vi "crio_FPGA_encoder.vi"() -> ()   [LabVIEW 2019]
uses:
  <vilib>/rvi/Emulation/niFpgaSctlEmulationGetInTimedLoop.vi
  <vilib>/rvi/Emulation/niFpgaProcessEmulError.vi
  <vilib>/rvi/eio/common/nirviEmuTemplateMethod_errors.vi
  <vilib>/rvi/Emulation/niFpgaGetClockAttributes.vi
  <vilib>/rvi/Emulation/niFpgaEmulationReportErrorSimple.vi
  <vilib>/rvi/Emulation/niFpgaCriticalErrorInLSC.vi
  <vilib>/eio/EIOMethodNode/EIOMethodNode.xnode
  <vilib>/eio/EIONode/EIONode.xnode
panel:
  in  "stop":bool
  in  "Encoder Debug":bool
  in  "Loop Timer DAQ":u32=1 caption="Loop Time(uSec)"
  in  "Position Reset":bool
  out "Position (Counts)":i64
  out "B":bool
  out "A":bool
  out "B'":bool
  out "A'":bool
  in  "Velocity Interval (uSec)":u32=1000
  out "Acceleration (Counts/Interval)":i32
  out "Velocity (Counts/Interval)":i32
  out "ConnectorA/DIO13":bool
  out "ConnectorA/DIO12":bool
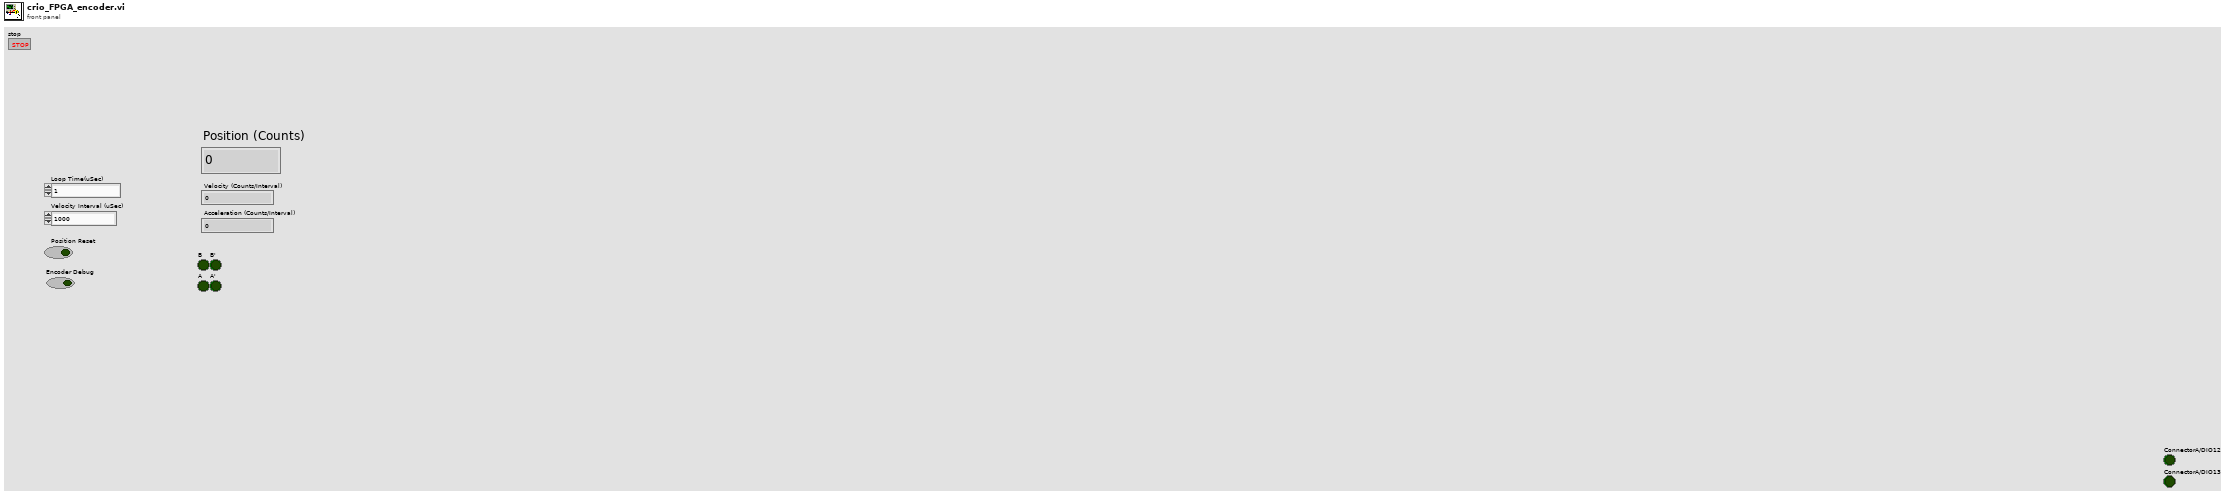
[diagram p1: front panel]
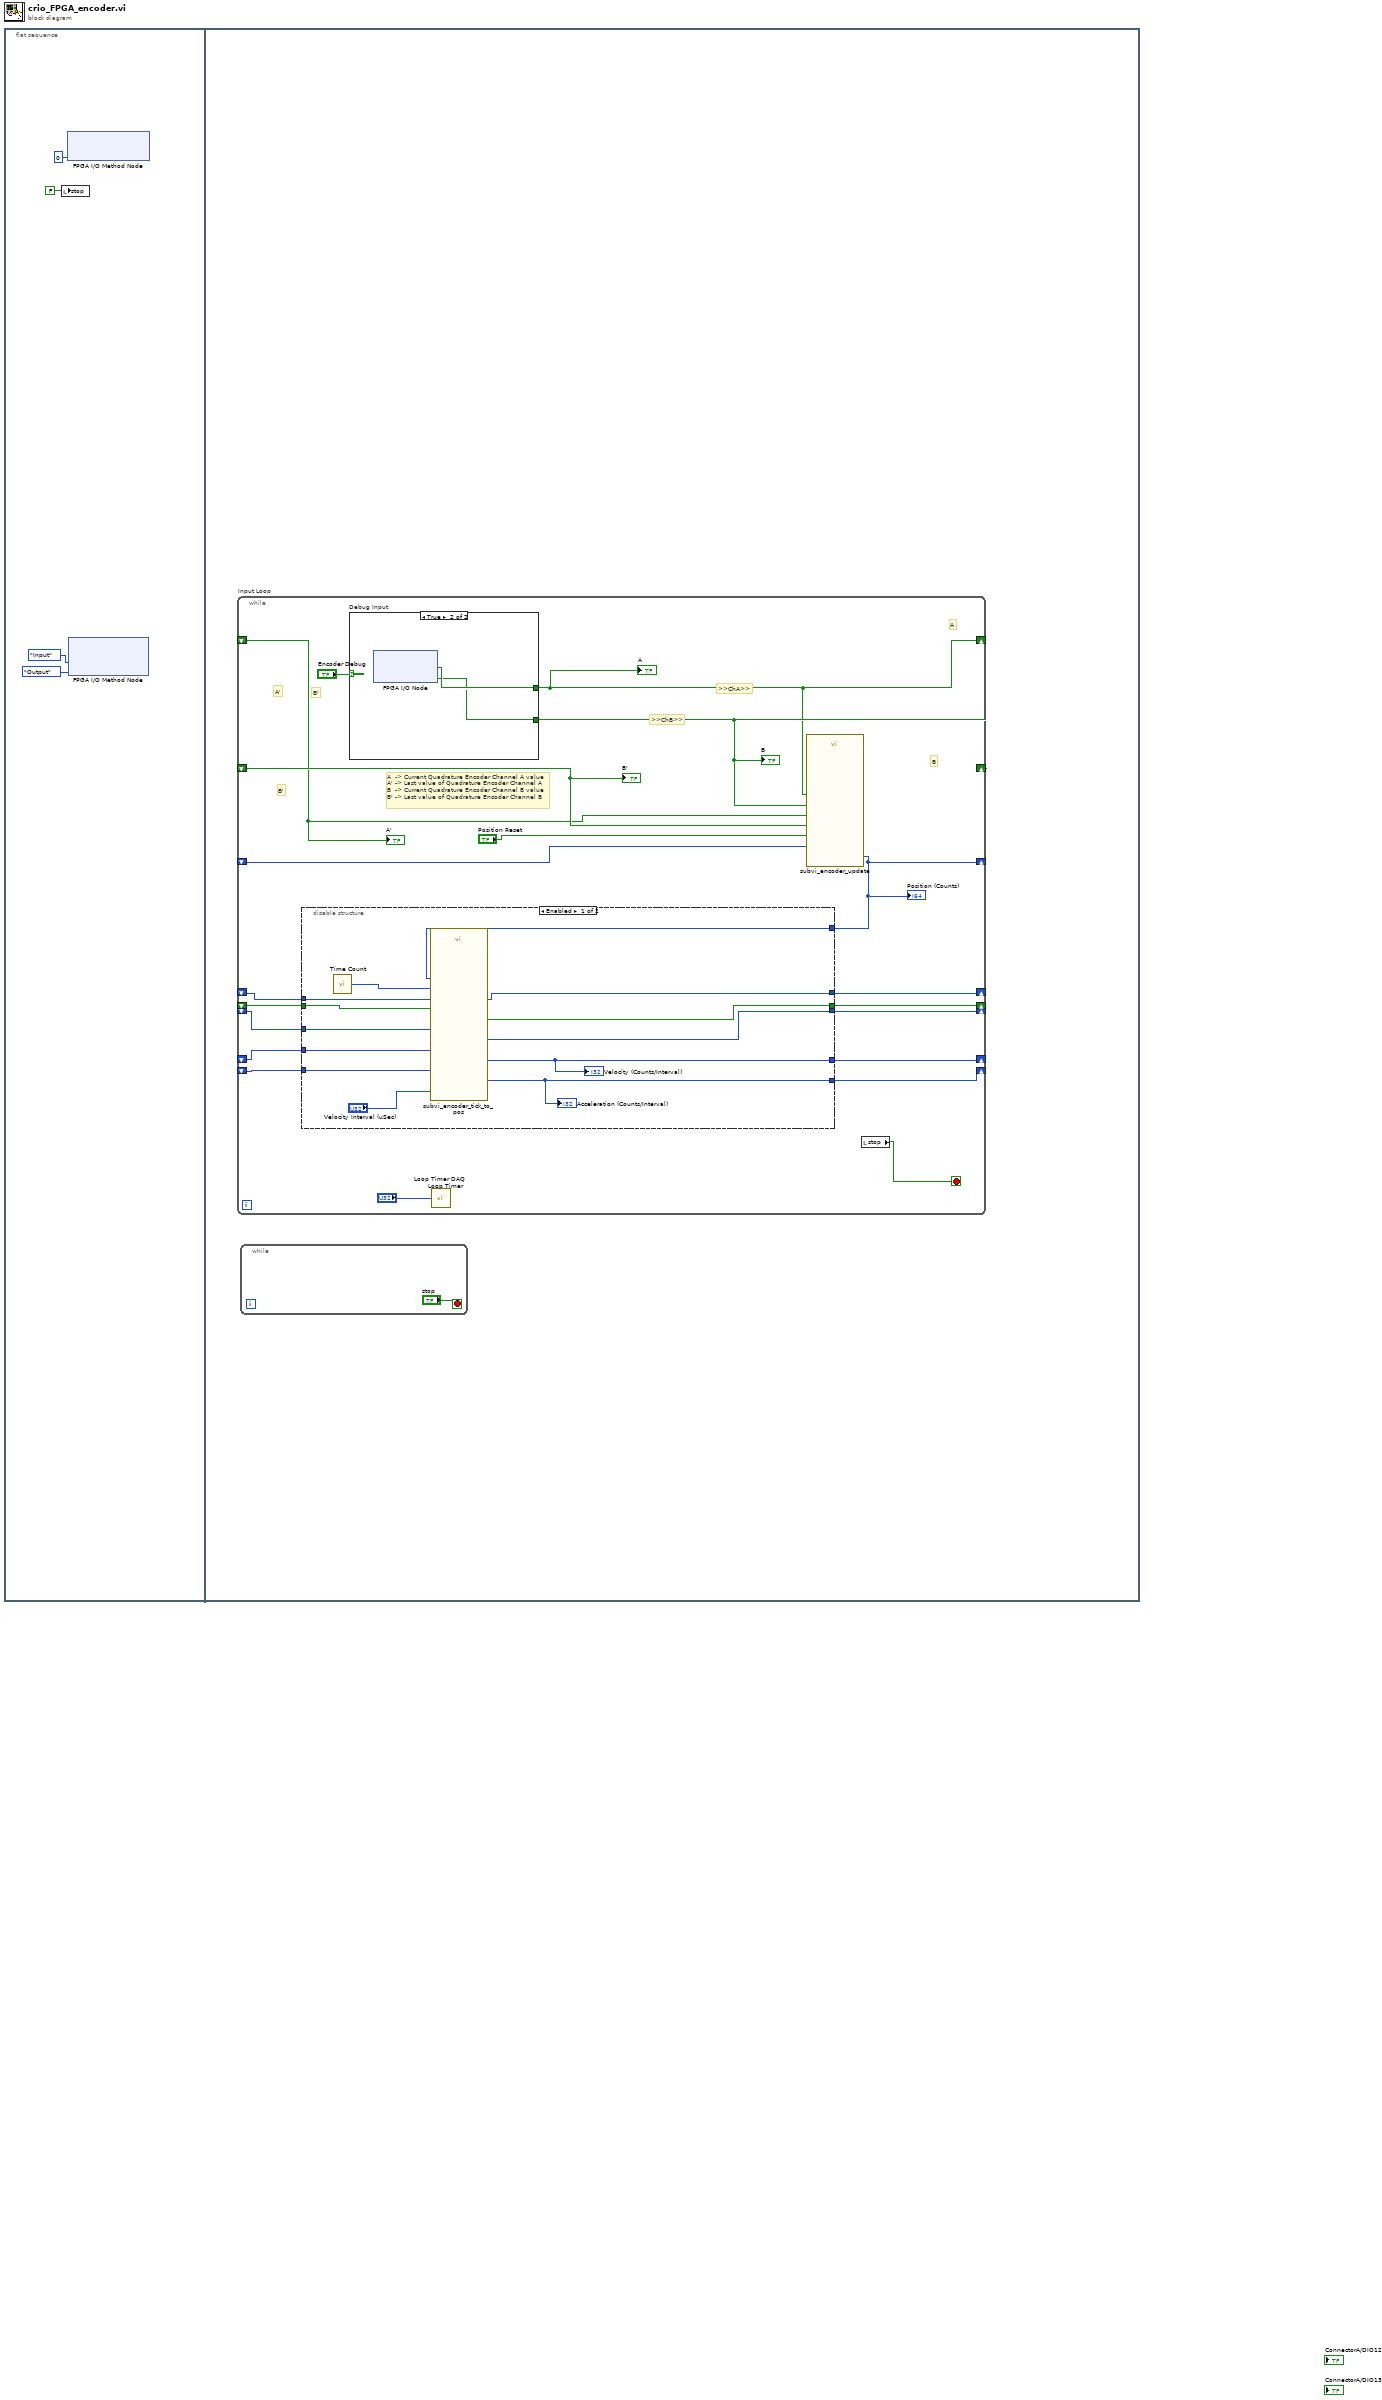
[diagram p0: block diagram]
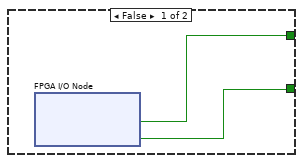
[diagram p3: hidden frame]
diagram:
  n1 = flat-sequence {
    frame #0 {
      n2 = local write "stop"(FALSE ("stop")) -> ()
      n3 = xnode "FPGA I/O Method Node"("Enable"=u8 0) -> ()  [unwired: 1 in, 1 out]
      n4 = xnode "FPGA I/O Method Node"("DIO 7:4"=enum8{"No Change", "Input", "Output"}."Input", "DIO 3:0"=enum8{"No Change", "Input", "Output"}."Output") -> ()  [unwired: 1 in, 1 out]
    }
    frame #1 {
      n5 = while "Input Loop" {
        shift-right: [w19] -> _
        shift-left: _ -> [w22]
        shift-right: [w18] -> _
        shift-left: _ -> [w21]
        shift-right: [w14] -> _
        shift-left: _ -> [w20]
        shift-right: [w7] -> _
        shift-left: _ -> [w17]
        shift-right: [w8] -> _
        shift-left: _ -> [w16]
        shift-right: [w15] -> _
        shift-left: _ -> [w13]
        shift-right: [w12] -> _
        shift-left: _ -> [w11]
        shift-right: [w10] -> _
        shift-left: _ -> [w9]
        stop <- w6 stop-if-true
        # "B'"
        # ">>ChB>>"
        # ">>ChA>>"
        # "A'"
        # "A  -> Current Quadrature Encoder Channel A value\nA' -> Last value of Quadrature Encoder Channel A\nB  -> Current Quadrature Encoder Channel B value\nB' -> Last value of Quadrature Encoder Channel B"
        # "B'"
        # "B"
        # "A"
        n6 = case "Debug Input" shown="True" "Encoder Debug" {
          tunnel: [w40 w42] -> w18
          tunnel: [w39 w41] -> w19
          frame False {
            n7 = xnode "FPGA I/O Node"() -> ("Mod2/DIO0"=w40:bool, "Mod2/DIO1"=w39:bool)  [unwired: 2 in, 2 out]
          }
          frame True {
            n8 = xnode "FPGA I/O Node"() -> ("Mod1/DIO4"=w42:bool, "Mod1/DIO5"=w41:bool)  [unwired: 2 in, 2 out]
          }
        }
        "B" <- w19
        "A" <- w18
        n9 = call "Loop Timer"("Count(uSec)"="Loop Timer DAQ") -> ()  [unwired: 1 out]
        n10 = call "subvi_encoder_update.vi"("Position Reset"="Position Reset", "Tick'"=w20, "A"=w18, "B'"=w22, "A'"=w21, "B"=w19) -> ("Tick"=w14:i32)  [unwired: 5 in]
        "Position (Counts)" <- w14
        n11 = disable-structure shown="Enabled" {
          disable-tunnel: w17 -> [w37 _]
          disable-tunnel: w16 -> [w36 _]
          disable-tunnel: [w35 _] -> w15
          disable-tunnel: w14 -> [w34 _]
          disable-tunnel: w13 -> [w33 _]
          disable-tunnel: [w32 _] -> w12
          disable-tunnel: w11 -> [w31 _]
          disable-tunnel: [w30 _] -> w10
          disable-tunnel: w9 -> [w29 _]
          disable-tunnel: [w27 _] -> w8
          disable-tunnel: [w26 _] -> w7
          frame Enabled {
            n12 = call "Time Count"() -> ("Tick Count(uSec)"=w28:u32)
            n13 = call "subvi_encoder_tick_to_pos.vi"("Velocity Interval (uSec)"="Velocity Interval (uSec)", "Raw Tick"=w34, "Waited?'"=w31, "Tick Count(uSec)'"=w29, "p'"=w33, "Time Count"=w28, "a'"=w36, "v'"=w37) -> ("Waited?"=w32:bool, "Tick Count(uSec)"=w30:u32, "p"=w35:i32, "a"=w27:i32, "v"=w26:i32)  [unwired: 3 in]
            "Acceleration (Counts/Interval)" <- w27
            "Velocity (Counts/Interval)" <- w26
          }
          frame Disabled {
          }
        }
        n14 = local read "stop"() -> (w6:bool)
        "B'" <- w22
        "A'" <- w21
      }
      n15 = while {
        stop <- "stop" stop-if-true
      }
    }
  }
